vi "ConvertRectangularROI2AnnularROI.vi"(8 "error in (no error)":errorcluster, 11 "ROI":T1) -> (0 "error out":errorcluster, 3 "Annulus":T2 {"End Angle" min=-90.0 max=90.0 step=1.0 format="%.2f"; "Start Angle" min=-90.0 max=90.0 step=1.0 format="%.2f"; "Center X" scale=0.0..1024.0})   [LabVIEW 2019, in "Algorithm.lvclass"]
uses:
  FrameworkOverrides/Algorithm.lvclass
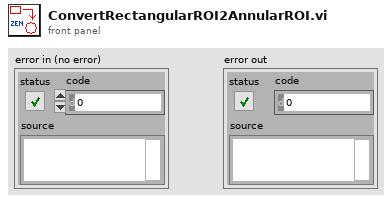
[diagram p1: front panel]
types:
  T1 = cluster{"Global Rectangle":i32[], "Contours":cluster{"Contour Type":u32, "ROI Type":u32, "Points":i32[]}[]}
  T2 = typedef "IMAQ Circle" = cluster{"Center X":i32, "Center Y":i32, "Inner Radius":i32, "Outer Radius":i32, "Start Angle":dbl, "End Angle":dbl}
  T3 = typedef "IMAQ Rectangle" = cluster{"Left":i32, "Top":i32, "Right":i32, "Bottom":i32, "Rotation":dbl}
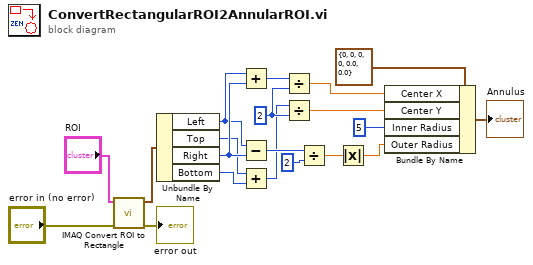
[diagram p0: block diagram]
diagram:
  w8 = 2
  n1 = call "IMAQ Convert ROI to Rectangle"("error in (no error)"="error in (no error)", "ROI Descriptor"="ROI") -> ("error out"=→"error out":errorcluster, "Rectangle"=w3:T3)  [unwired: 7 in]
  n2 = Unbundle By Name(w3) -> ("Left"=w13:i32, "Top"=w4:i32, "Right"=w14:i32, "Bottom"=w5:i32)
  n3 = Add(x=w13, y=w14) -> (x+y=w6:i32)
  n4 = Subtract(x=w13, y=w14) -> (x-y=w16:i32)
  n5 = Add(x=w4, y=w5) -> (x+y=w7:i32)
  n6 = Divide(x=w6, y=w8) -> (x/y=w10:dbl)
  n7 = Divide(x=w7, y=w8) -> (x/y=w11:dbl)
  n8 = Divide(x=w16, y=2) -> (x/y=w17:dbl)
  n9 = Absolute Value(x=w17) -> (abs(x)=w18:dbl)
  n10 = Bundle By Name(cluster=T2 {"Center X"=0, "Center Y"=0, "Inner Radius"=0, "Outer Radius"=0, "Start Angle"=0.0, "End Angle"=0.0} ("Annulus"), "Center X"=w10, "Center Y"=w11, "Inner Radius"=5, "Outer Radius"=w18) -> (→"Annulus":T2)
